vi "MV main 1.5.vi"() -> ()   [LabVIEW 2015, in "Millennia V.lvclass"]
uses:
  Millennia V.lvclass
  MV status.ctl
  MV warmed up.ctl
  MV state.ctl
  MV warm-up state.ctl
panel:
  out "status indicators":T1 {"Warmed up" scale=0.0..100.0}
  in  "setpower":bool
  in  "power ctrl":dbl=0.2 min=0.2 max=5.0 step=0.01 format="%.2g"
  out "Power (W)":dbl(knob) scale=0.0..5.0
  in  "exit":bool
  in  "warm-up/on":bool
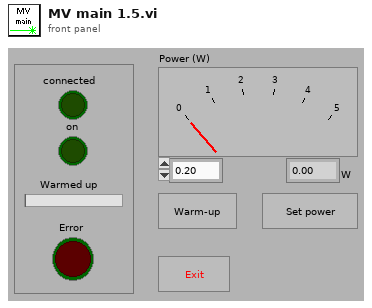
[diagram p1: front panel]
types:
  T1 = typedef "Millennia V.lvclass/MV status.ctl" = cluster{"Millennia V found":bool, "on?":bool, "Error":bool, "Warmed up":T2}
  T2 = typedef "Millennia V.lvclass/MV warmed up.ctl" = dbl
  T3 = typedef "Millennia V.lvclass/MV state.ctl" = enum16{"warm up", "turn on", "set power", "turn off", "end"}
  T4 = typedef "Millennia V.lvclass/MV warm-up state.ctl" = enum16{"read progress", "wait", "done"}
  T5 = enum16{"read only", "write only", "write + read"}
  T6 = cluster{"command error":bool, "execution error":bool, "system error":bool, "laser on":bool, "error":bool, "reserved 1":bool, "reserved 2":bool, "reserved 3":bool}
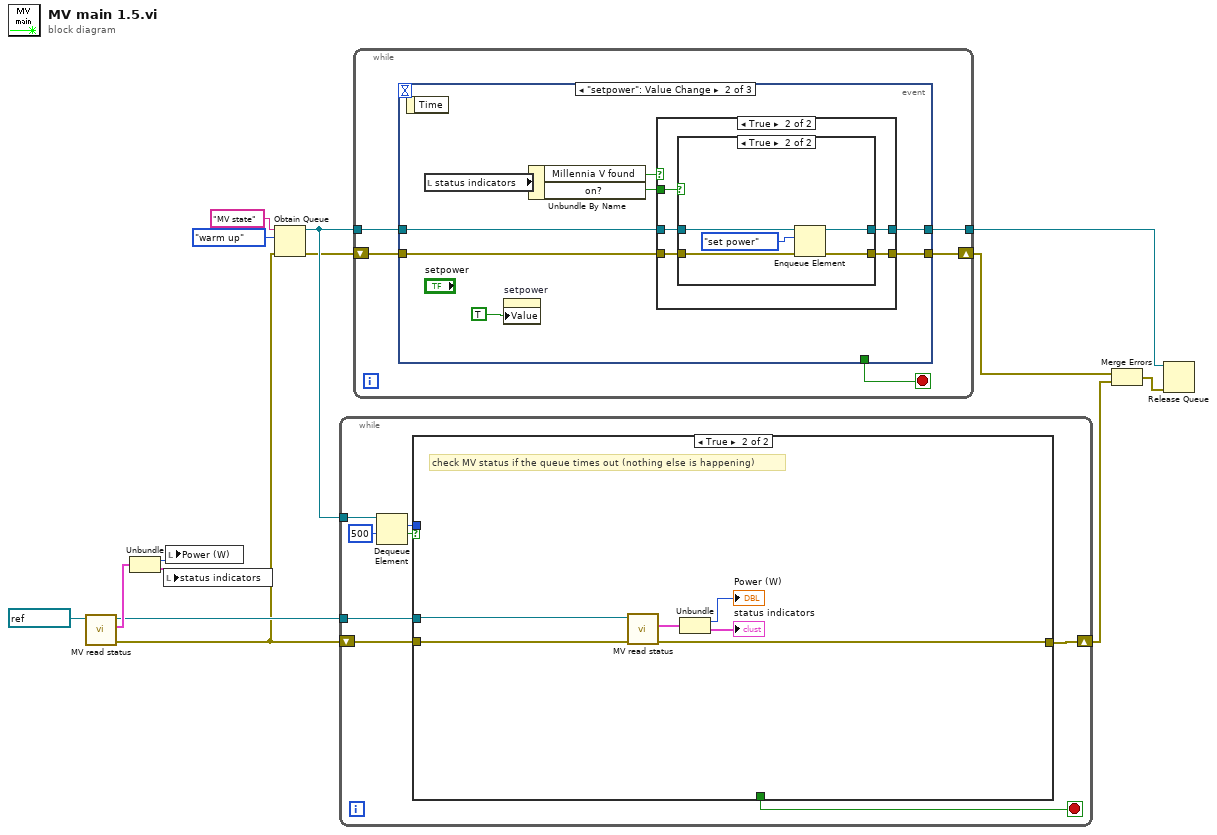
[diagram p0: block diagram]
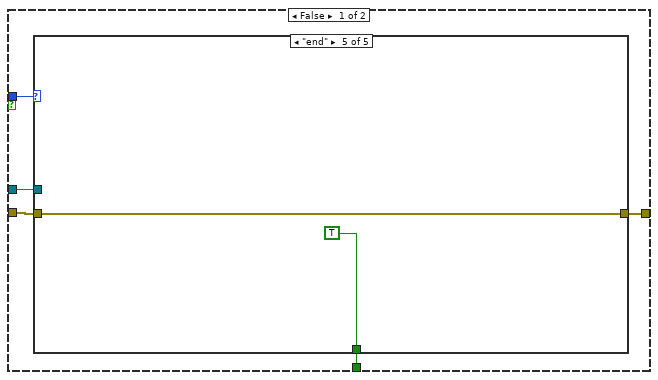
[diagram p2: hidden frame]
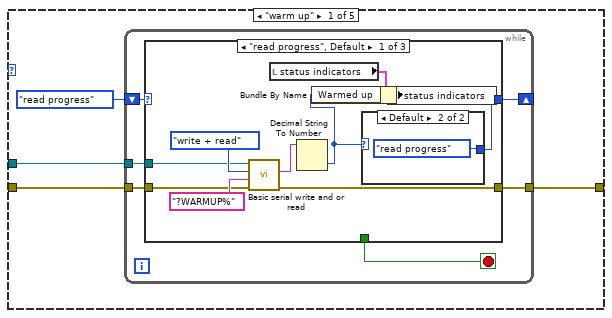
[diagram p3: hidden frame]
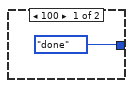
[diagram p4: hidden frame]
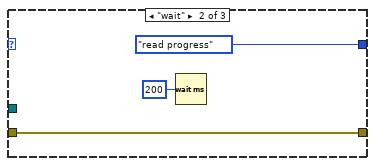
[diagram p5: hidden frame]
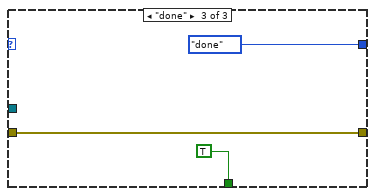
[diagram p6: hidden frame]
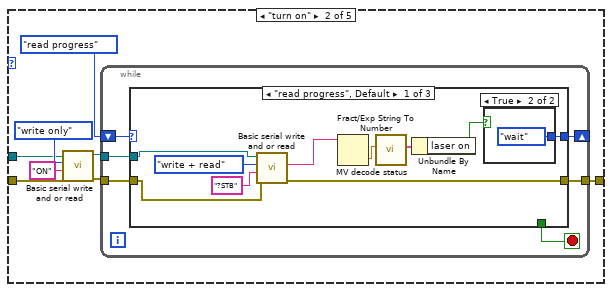
[diagram p7: hidden frame]
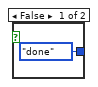
[diagram p8: hidden frame]
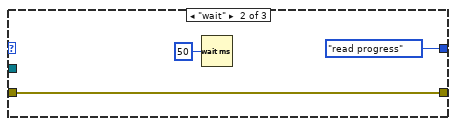
[diagram p9: hidden frame]
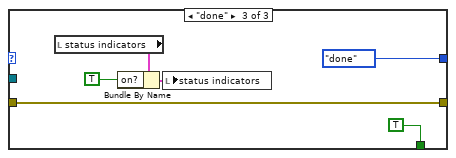
[diagram p10: hidden frame]
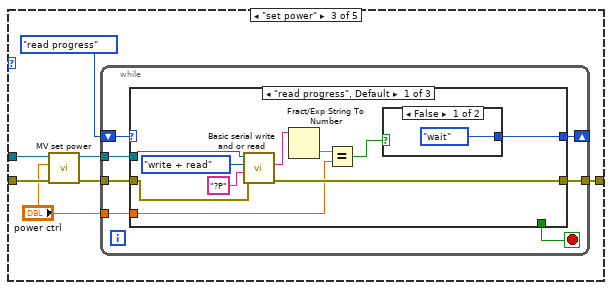
[diagram p11: hidden frame]
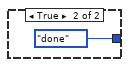
[diagram p12: hidden frame]
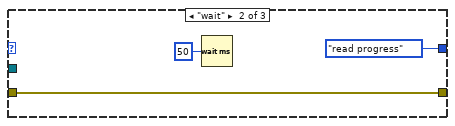
[diagram p13: hidden frame]
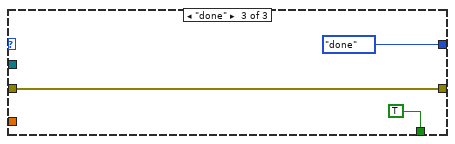
[diagram p14: hidden frame]
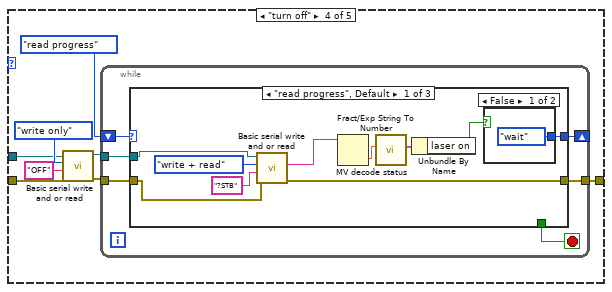
[diagram p15: hidden frame]
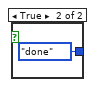
[diagram p16: hidden frame]
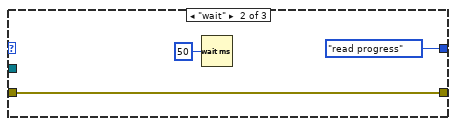
[diagram p17: hidden frame]
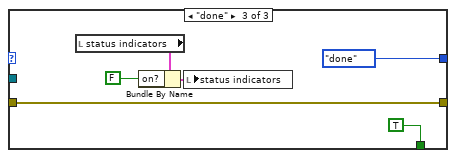
[diagram p18: hidden frame]
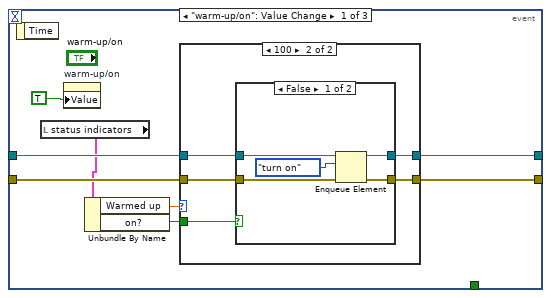
[diagram p19: hidden frame]
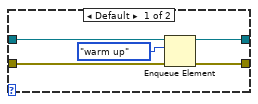
[diagram p20: hidden frame]
diagram:
  n1 = call "MV read status.vi"("VISA resource name"=refnum<visa-resource-name> "COM1") -> ("error out"=w6:errorcluster, "status cluster"=w10:cluster{"Power (W)":i32, "status indicators":T1}, "VISA resource name out"=w7:refnum<visa-resource-name>)  [unwired: 8 in]
  n2 = Unbundle(w10) -> ("Power (W)"=w9:i32, "status indicators"=w5:T1)
  n3 = local write "status indicators"(w5) -> ()
  n4 = local write "Power (W)"(w9) -> ()
  n5 = Obtain Queue(name (unnamed)="MV state", element data type=MV_state."warm up" ("Millennia state"), error in (no error)=w6) -> (queue out=w12:refnum<queue>, error out=w11:errorcluster)  [unwired: 2 in, 1 out]
  n6 = while {
    tunnel: w12 -> [w22]
    shift-right: [w16] -> w3
    shift-left: w6 -> [w20]
    tunnel: w7 -> [w19]
    stop <- w18 stop-if-true
    n7 = Dequeue Element(queue=w22, timeout in ms (-1)=500) -> (element=w21:T3, timed out?=w17:bool)  [unwired: 1 in, 2 out]
    n8 = case shown="True" w17 {
      tunnel: w21 -> [w27 _]
      tunnel: w20 -> [w26 w162]
      tunnel: w19 -> [w25 w163]
      tunnel: [w24 _] -> w18
      tunnel: [w23 w161] -> w16
      frame False {
        n9 = case shown="\"end\"" w27 {
          tunnel: w26 -> [w30 w58 w93 w125 w158]
          tunnel: w25 -> [w31 w60 w95 w127 _]
          tunnel: [_ _ _ _ TRUE] -> w24
          tunnel: [w29 w63 w97 w130 w158] -> w23
          frame "warm up" {
            n10 = while {
              tunnel: w31 -> [w37]
              tunnel: w30 -> [w36]
              tunnel: [w35] -> w29
              shift-right: [w34] -> _
              shift-left: MV_warm-up_state."read progress" ("warmup state") -> [w33]
              stop <- w32 stop-if-true
              n11 = case shown="\"read progress\", Default" w33 {
                tunnel: w37 -> [w44 _ _]
                tunnel: w36 -> [w43 w50 w53]
                tunnel: [w42 w50 w53] -> w35
                tunnel: [w41 MV_warm-up_state."read progress" ("warmup state") MV_warm-up_state."done" ("warmup state")] -> w34
                tunnel: [_ _ TRUE] -> w32
                frame "read progress", Default {
                  n12 = call "Basic serial write and or read.vi"("error in (no error)"=w43, "write string"="?WARMUP%", "action"=T5."write + read", "VISA resource name"=w44) -> ("error out"=w42:errorcluster, "read string"=w47:string)  [unwired: 4 in, 2 out]
                  n13 = local read "status indicators"() -> (w40:T1)
                  n14 = Decimal String To Number(string=w47) -> (number=w38:i32)  [unwired: 2 in, 1 out]
                  n15 = Bundle By Name(cluster=w40, "Warmed up"=w38) -> (w39:T1)
                  n16 = case shown="Default" w38 {
                    tunnel: [MV_warm-up_state."done" ("warmup state") MV_warm-up_state."read progress" ("warmup state")] -> w41
                    frame 100 {
                    }
                    frame Default {
                    }
                  }
                  n17 = local write "status indicators"(w39) -> ()
                }
                frame "wait" {
                  n18 = Wait (ms)(milliseconds to wait=u32 200) -> ()  [unwired: 1 out]
                }
                frame "done" {
                }
              }
            }
          }
          frame "turn on" {
            n19 = call "Basic serial write and or read.vi"("error in (no error)"=w58, "write string"="ON", "action"=T5."write only", "VISA resource name"=w60) -> ("error out"=w57:errorcluster, "VISA resource name out"=w59:refnum<visa-resource-name>)  [unwired: 4 in, 2 out]
            n20 = while {
              tunnel: w59 -> [w69]
              tunnel: w57 -> [w68]
              tunnel: [w67] -> w63
              shift-right: [w66] -> _
              shift-left: MV_warm-up_state."read progress" ("warmup state") -> [w65]
              stop <- w64 stop-if-true
              n21 = case shown="\"read progress\", Default" w65 {
                tunnel: w69 -> [w75 _ _]
                tunnel: w68 -> [w76 w84 w89]
                tunnel: [w77 w84 w89] -> w67
                tunnel: [w70 MV_warm-up_state."read progress" ("warmup state") MV_warm-up_state."done" ("warmup state")] -> w66
                tunnel: [_ _ TRUE] -> w64
                frame "read progress", Default {
                  n22 = call "Basic serial write and or read.vi"("error in (no error)"=w76, "write string"="?STB", "action"=T5."write + read", "VISA resource name"=w75) -> ("error out"=w77:errorcluster, "read string"=w73:string)  [unwired: 4 in, 2 out]
                  n23 = Fract/Exp String To Number(string=w73) -> (number=w72:dbl)  [unwired: 3 in, 1 out]
                  n24 = call "MV decode status.vi"("status byte"=w72) -> ("status cluster"=w74:T6)  [unwired: 10 in]
                  n25 = Unbundle By Name(w74) -> ("laser on"=w71:bool)
                  n26 = case shown="True" w71 {
                    tunnel: [MV_warm-up_state."done" ("warmup state") MV_warm-up_state."wait" ("warmup state")] -> w70
                    frame False {
                    }
                    frame True {
                    }
                  }
                }
                frame "wait" {
                  n27 = Wait (ms)(milliseconds to wait=u32 50) -> ()  [unwired: 1 out]
                }
                frame "done" {
                  n28 = local read "status indicators"() -> (w87:T1)
                  n29 = Bundle By Name(cluster=w87, "on?"=TRUE) -> (w85:T1)
                  n30 = local write "status indicators"(w85) -> ()
                }
              }
            }
          }
          frame "set power" {
            n31 = call "MV set power.vi"("error in (no error)"=w93, "power (W)"="power ctrl", "VISA resource name"=w95) -> ("error out"=w92:errorcluster, "VISA resource name out"=w94:refnum<visa-resource-name>)  [unwired: 7 in]
            n32 = while {
              tunnel: w94 -> [w104]
              tunnel: w92 -> [w103]
              tunnel: [w102] -> w97
              shift-right: [w101] -> _
              shift-left: MV_warm-up_state."read progress" ("warmup state") -> [w100]
              tunnel: "power ctrl" -> [w98]
              stop <- w99 stop-if-true
              n33 = case shown="\"read progress\", Default" w100 {
                tunnel: w104 -> [w110 _ _]
                tunnel: w103 -> [w111 w119 w121]
                tunnel: [w112 w119 w121] -> w102
                tunnel: [w108 MV_warm-up_state."read progress" ("warmup state") MV_warm-up_state."done" ("warmup state")] -> w101
                tunnel: [_ _ TRUE] -> w99
                tunnel: w98 -> [w106 _ _]
                frame "read progress", Default {
                  n34 = call "Basic serial write and or read.vi"("error in (no error)"=w111, "write string"="?P", "action"=T5."write + read", "VISA resource name"=w110) -> ("error out"=w112:errorcluster, "read string"=w109:string)  [unwired: 4 in, 2 out]
                  n35 = Fract/Exp String To Number(string=w109) -> (number=w107:dbl)  [unwired: 3 in, 1 out]
                  n36 = Equal?(x=w107, y=w106) -> (x = y?=w105:bool)
                  n37 = case shown="False" w105 {
                    tunnel: [MV_warm-up_state."wait" ("warmup state") MV_warm-up_state."done" ("warmup state")] -> w108
                    frame False {
                    }
                    frame True {
                    }
                  }
                }
                frame "wait" {
                  n38 = Wait (ms)(milliseconds to wait=u32 50) -> ()  [unwired: 1 out]
                }
                frame "done" {
                }
              }
            }
          }
          frame "turn off" {
            n39 = call "Basic serial write and or read.vi"("error in (no error)"=w125, "write string"="OFF", "action"=T5."write only", "VISA resource name"=w127) -> ("error out"=w124:errorcluster, "VISA resource name out"=w126:refnum<visa-resource-name>)  [unwired: 4 in, 2 out]
            n40 = while {
              tunnel: w126 -> [w136]
              tunnel: w124 -> [w135]
              tunnel: [w134] -> w130
              shift-right: [w133] -> _
              shift-left: MV_warm-up_state."read progress" ("warmup state") -> [w132]
              stop <- w131 stop-if-true
              n41 = case shown="\"read progress\", Default" w132 {
                tunnel: w136 -> [w142 _ _]
                tunnel: w135 -> [w143 w151 w156]
                tunnel: [w144 w151 w156] -> w134
                tunnel: [w137 MV_warm-up_state."read progress" ("warmup state") MV_warm-up_state."done" ("warmup state")] -> w133
                tunnel: [_ _ TRUE] -> w131
                frame "read progress", Default {
                  n42 = call "Basic serial write and or read.vi"("error in (no error)"=w143, "write string"="?STB", "action"=T5."write + read", "VISA resource name"=w142) -> ("error out"=w144:errorcluster, "read string"=w140:string)  [unwired: 4 in, 2 out]
                  n43 = Fract/Exp String To Number(string=w140) -> (number=w139:dbl)  [unwired: 3 in, 1 out]
                  n44 = call "MV decode status.vi"("status byte"=w139) -> ("status cluster"=w141:T6)  [unwired: 10 in]
                  n45 = Unbundle By Name(w141) -> ("laser on"=w138:bool)
                  n46 = case shown="False" w138 {
                    tunnel: [MV_warm-up_state."wait" ("warmup state") MV_warm-up_state."done" ("warmup state")] -> w137
                    frame False {
                    }
                    frame True {
                    }
                  }
                }
                frame "wait" {
                  n47 = Wait (ms)(milliseconds to wait=u32 50) -> ()  [unwired: 1 out]
                }
                frame "done" {
                  n48 = local read "status indicators"() -> (w154:T1)
                  n49 = Bundle By Name(cluster=w154, "on?"=FALSE) -> (w152:T1)
                  n50 = local write "status indicators"(w152) -> ()
                }
              }
            }
          }
          frame "end" {
          }
        }
      }
      frame True {
        # "check MV status if the queue times out (nothing else is happening)"
        n51 = call "MV read status.vi"("error in (no error)"=w162, "VISA resource name"=w163) -> ("error out"=w161:errorcluster, "status cluster"=w164:cluster{"Power (W)":i32, "status indicators":T1})  [unwired: 7 in, 1 out]
        n52 = Unbundle(w164) -> ("Power (W)"=→"Power (W)":i32, "status indicators"=→"status indicators":T1)
      }
    }
  }
  n53 = while {
    tunnel: w12 -> [w169]
    shift-right: [w167] -> w4
    shift-left: w11 -> [w168]
    tunnel: [w166] -> w2
    stop <- w170 stop-if-true
    n54 = event shown="[1] \"setpower\": Value Change" {
      selector: _ -> [_ _ _]
      dyn-events: _ -> [_ _ _]
      timeout: _ -> [_ _ _]
      tunnel: [_ _ TRUE] -> w170
      tunnel: w169 -> [w178 w203 w227]
      tunnel: w168 -> [w177 w202 w226]
      tunnel: [w176 w201 w225] -> w167
      tunnel: [w172 w200 w224] -> w166
      event "warm-up/on": Value Change {
        n55 = event-data() -> ()  [unwired: 1 in, 1 out]
        n56 = local read "status indicators"() -> (w175:T1)
        n57 = property on="warm-up/on" class="Bool (strict)"("Value"=TRUE ("warm-up/on")) -> ()  [unwired: 2 in, 2 out]
        n58 = Unbundle By Name(w175) -> ("Warmed up"=w174:T2, "on?"=w173:bool)
        n59 = case shown="100" w174 {
          tunnel: w178 -> [w183 w188]
          tunnel: w177 -> [w182 w187]
          tunnel: [w181 w186] -> w176
          tunnel: w173 -> [_ w185]
          tunnel: [w179 w184] -> w172
          frame Default {
            n60 = Enqueue Element(queue=w183, element=MV_state."warm up" ("Millennia state"), error in (no error)=w182) -> (queue out=w179:refnum<queue>, error out=w181:errorcluster)  [unwired: 1 in, 1 out]
          }
          frame 100 {
            n61 = case shown="False" w185 {
              tunnel: w188 -> [w193 w198]
              tunnel: w187 -> [w191 w196]
              tunnel: [w190 w195] -> w186
              tunnel: [w189 w194] -> w184
              frame False {
                n62 = Enqueue Element(queue=w193, element=MV_state."turn on" ("Millennia state"), error in (no error)=w191) -> (queue out=w189:refnum<queue>, error out=w190:errorcluster)  [unwired: 1 in, 1 out]
              }
              frame True {
                n63 = Enqueue Element(queue=w198, element=MV_state."turn off" ("Millennia state"), error in (no error)=w196) -> (queue out=w194:refnum<queue>, error out=w195:errorcluster)  [unwired: 1 in, 1 out]
              }
            }
          }
        }
      }
      event "setpower": Value Change {
        n64 = event-data() -> ()  [unwired: 1 in, 1 out]
        n65 = local read "status indicators"() -> (w206:T1)
        n66 = property on="setpower" class="Bool (strict)"("Value"=TRUE ("setpower")) -> ()  [unwired: 2 in, 2 out]
        n67 = Unbundle By Name(w206) -> ("Millennia V found"=w205:bool, "on?"=w204:bool)
        n68 = case shown="True" w205 {
          tunnel: w204 -> [_ w214]
          tunnel: w203 -> [w207 w213]
          tunnel: w202 -> [w208 w212]
          tunnel: [w208 w211] -> w201
          tunnel: [w207 w210] -> w200
          frame False {
            n69 = One Button Dialog(message="Millennia V laser not found. Please check connections and try again.") -> ()  [unwired: 1 in, 1 out]
          }
          frame True {
            n70 = case shown="True" w214 {
              tunnel: w213 -> [w215 w221]
              tunnel: w212 -> [w216 w220]
              tunnel: [w216 w219] -> w211
              tunnel: [w215 w218] -> w210
              frame False {
                n71 = One Button Dialog(message="The Millennia V laser is not fully powered on. Please turn it on before setting the power.") -> ()  [unwired: 1 in, 1 out]
              }
              frame True {
                n72 = Enqueue Element(queue=w221, element=MV_state."set power" ("Millennia state"), error in (no error)=w220) -> (queue out=w218:refnum<queue>, error out=w219:errorcluster)  [unwired: 1 in, 1 out]
              }
            }
          }
        }
      }
      event "exit": Value Change; Application Instance Close; Panel Close {
        n73 = event-data() -> ()  [unwired: 1 in, 1 out]
        n74 = property on="exit" class="Bool (strict)"("Value"=FALSE ("exit")) -> ()  [unwired: 2 in, 2 out]
        n75 = Enqueue Element(queue=w227, element=MV_state."end" ("Millennia state"), error in (no error)=w226) -> (queue out=w224:refnum<queue>, error out=w225:errorcluster)  [unwired: 1 in, 1 out]
      }
    }
  }
  n76 = Merge Errors(w4, w3) -> (w1:errorcluster)
  n77 = Release Queue(queue=w2, error in (no error)=w1) -> ()  [unwired: 1 in, 3 out]
